vi "Day 4.1 - Bingo.vi"(9 "bingo cards":i32[][][](array[numeric]), 11 "bingo calls":i32[](array[numeric])) -> (3 "output":u32)   [LabVIEW 2021]
panel:
  out "Winning Card":i32
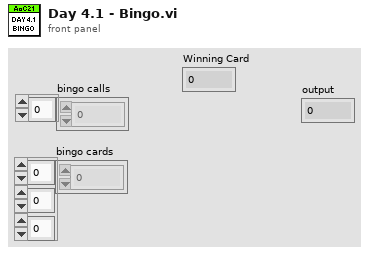
[diagram p1: front panel]
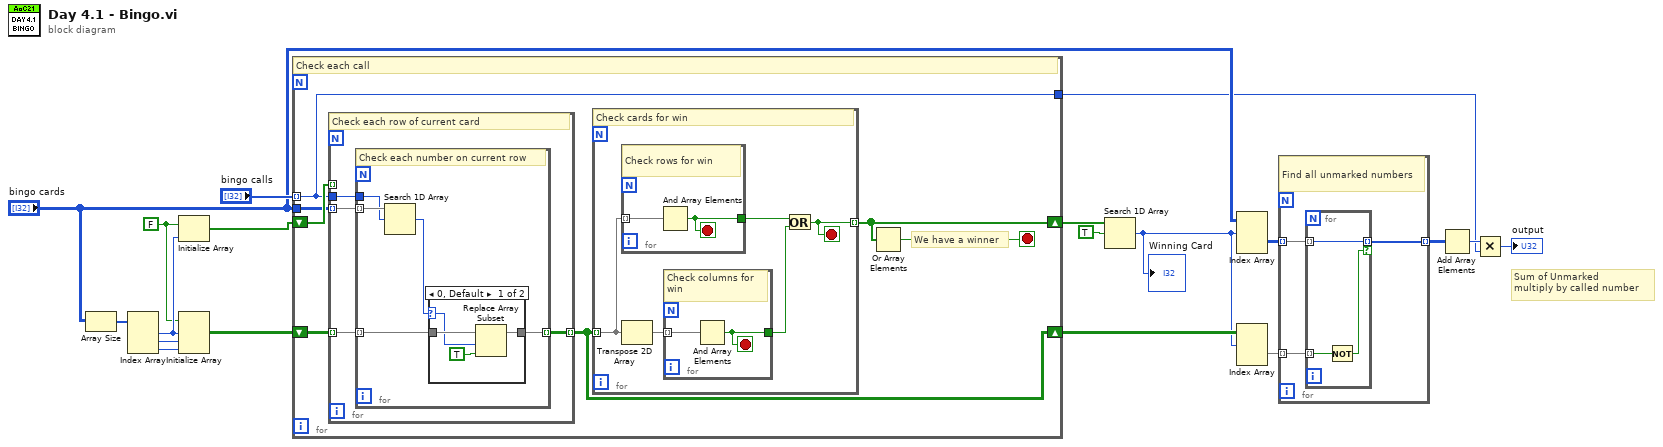
[diagram p0: block diagram]
diagram:
  w12 = FALSE
  # "Sum of Unmarked\nmultiply by called number"
  n1 = Array Size(array="bingo cards") -> (size(s)=w18:i32[])
  n2 = Index Array(array=w18) -> (element #1=w13:i32, element #2=w17:i32, element #3=w16:i32)  [unwired: 3 in]
  n3 = Initialize Array(w12, w13) -> (w14:bool[])
  n4 = Initialize Array(w12, w13, w17, w16) -> (w15:bool[][][])
  n5 = for {
    tunnel: "bingo calls" -> [w20] mode=indexing
    shift-right: [w24] -> w8
    shift-left: w15 -> [w26]
    shift-right: [w22] -> w11
    shift-left: w14 -> [w25]
    tunnel: "bingo cards" -> [w23]
    tunnel: [w20] -> w1
    stop <- w21 stop-if-true
    # "We have a winner"
    # "Check each call"
    n6 = for {
      tunnel: w23 -> [w39] mode=indexing
      tunnel: w26 -> [w37] mode=indexing
      tunnel: w20 -> [w38]
      tunnel: w25 -> [_] mode=indexing
      tunnel: [w36] -> w24 mode=indexing
      # "Check each row of current card"
      n7 = for {
        tunnel: w39 -> [w44] mode=indexing
        tunnel: w38 -> [w43]
        tunnel: w37 -> [w41] mode=indexing
        tunnel: [w40] -> w36 mode=indexing
        # "Check each number on current row"
        n8 = Search 1D Array(1D array=w44, element=w43) -> (index of element=w42:i32)  [unwired: 1 in]
        n9 = case shown="0, Default" w42 {
          selector: w42 -> [w47 _]
          tunnel: [w45 w49] -> w40
          tunnel: w41 -> [w48 w49]
          frame 0, Default {
            n10 = Replace Array Subset(array=w48, new element=TRUE ("new element/subarray"), index=w47) -> (w45:bool[])
          }
          frame -1 {
          }
        }
      }
    }
    n11 = for {
      tunnel: w24 -> [w31] mode=indexing
      tunnel: [w27] -> w22 mode=indexing
      stop <- w27 stop-if-true
      # "Check cards for win"
      n12 = for {
        tunnel: w31 -> [w35] mode=indexing
        tunnel: [w34] -> w29
        stop <- w34 stop-if-true
        # "Check rows for win"
        n13 = And Array Elements(Boolean array=w35) -> (logical AND=w34:bool)
      }
      n14 = Transpose 2D Array(2D array=w31) -> (transposed array=w30:bool[][])
      n15 = for {
        tunnel: w30 -> [w33] mode=indexing
        tunnel: [w32] -> w28
        stop <- w32 stop-if-true
        # "Check columns for win"
        n16 = And Array Elements(Boolean array=w33) -> (logical AND=w32:bool)
      }
      n17 = Or(x=w29, y=w28) -> (x .or. y?=w27:bool)
    }
    n18 = Or Array Elements(Boolean array=w22) -> (logical OR=w21:bool)
  }
  n19 = Search 1D Array(1D array=w11, element=TRUE) -> (index of element=w7:i32)  [unwired: 1 in]
  "Winning Card" <- w7
  n20 = Index Array(array="bingo cards", index (dim 0)=w7) -> (element=w6:i32[][])  [unwired: 2 in]
  n21 = Index Array(array=w8, index (dim 0)=w7) -> (element=w5:bool[][])  [unwired: 2 in]
  n22 = for {
    tunnel: w6 -> [w52] mode=indexing
    tunnel: w5 -> [w51] mode=indexing
    tunnel: [w50] -> w4 mode=indexing
    # "Find all unmarked numbers"
    n23 = for {
      tunnel: w52 -> [w55] mode=indexing
      tunnel: w51 -> [w54] mode=indexing
      tunnel: [w55] -> w50 mode=indexing if=w53
      n24 = Not(x=w54) -> (.not. x?=w53:bool)
    }
  }
  n25 = Add Array Elements(numeric array=w4) -> (sum=w3:i32)
  n26 = Multiply(x=w3, y=w1) -> (x*y=→"output":i32)
